vi "Cluster Test.vi"() -> ()   [LabVIEW 2013]
panel:
  in  "?":bool
  out "Your password is:":string
  out "Your username is:":string
  in  "Test Cluster":cluster{"Username":string, "Password":string}
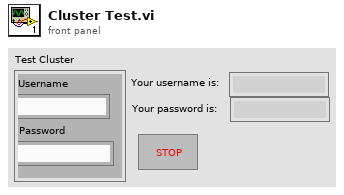
[diagram p1: front panel]
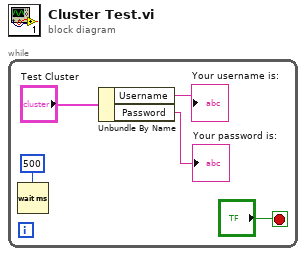
[diagram p0: block diagram]
diagram:
  n1 = while {
    stop <- "?" stop-if-true
    n2 = Wait (ms)(milliseconds to wait=u32 500) -> ()  [unwired: 1 out]
    n3 = Unbundle By Name("Test Cluster") -> ("Username"=→"Your username is:":string, "Password"=→"Your password is:":string)
  }
